vi "Mcp2210 Get Interrupt Count.vi"(8 "error in (no error)":errorcluster, 10 "Reset":bool, 11 "handle":i32) -> (0 "error out":errorcluster, 2 "pintCnt out":u32, 3 "handle out":i32)   [LabVIEW 2015, in "mcp2210.lvlib"]
doc: "Reads the event counter value. It may also reset the counter, depending on the reset\nparameter value. The function returns negative error code if something went wrong.\nNote: In order to have the MCP2210 record the number of external interrupt events,\nGP6 must be configured to have its dedicated function active.\nParameters:\nInputs:\n- void *handle - The pointer to the device handle. Cannot be NULL.\n- unsigned char reset - if set to 0, the counter is reset. Any other value has no effect.\nOutputs:\n- unsigned int *pintCnt - the value of the counter if the function returns E_SUCCESS.\nIn case of error *pintCnt is not modified.\nNote that the counter has 16bit resolution, so the maximum\nreturned value is 65535.\nCannot be NULL.\nReturns:\n- 0 for success: E_SUCCESS\n- negative error code: E_ERR_NULL, E_ERR_INVALID_HANDLE_VALUE\nE_ERR_UNKOWN_ERROR\nE_ERR_HID_TIMEOUT, E_ERR_HID_RW_FILEIO\nE_ERR_CMD_ECHO, E_ERR_CMD_FAILED\n\nMCP2210_DLL_UM_API int __stdcall Mcp2210_GetInterruptCount(void *handle, unsigned int *pintCnt, unsigned char reset);"
uses:
  <userlib>/mcp2210/mcp2210.lvlib
  <userlib>/mcp2210/mcp2210_dll_um_x86.dll
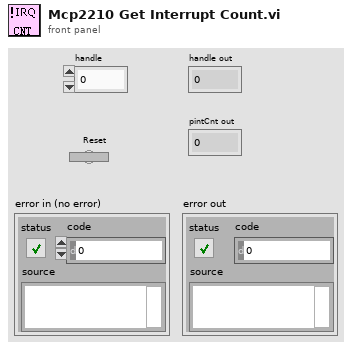
[diagram p1: front panel]
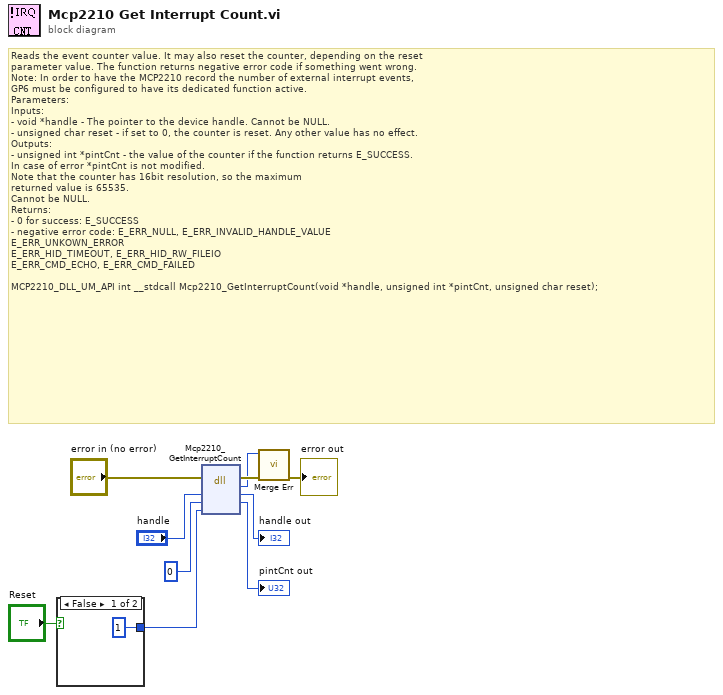
[diagram p0: block diagram]
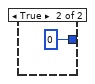
[diagram p2: hidden frame]
diagram:
  # "Reads the event counter value. It may also reset the counter, depending on the reset\nparameter value. The function returns negative error code if something went wrong.\nNote: In order to have the MCP2210 record the number of external interrupt events,\nGP6 must be configured to have its dedicated function active.\nParameters:\nInputs:\n- void *handle - The pointer to the device handle. Cannot be NULL.\n- unsigned char reset - if set to 0, the counter is reset. Any other value has no effect.\nOutputs:\n- unsigned int *pintCnt - the value of the counter if the function returns E_SUCCESS.\nIn case of error *pintCnt is not modified.\nNote that the counter has 16bit resolution, so the maximum\nreturned value is 65535.\nCannot be NULL.\nReturns:\n- 0 for success: E_SUCCESS\n- negative error code: E_ERR_NULL, E_ERR_INVALID_HANDLE_VALUE\nE_ERR_UNKOWN_ERROR\nE_ERR_HID_TIMEOUT, E_ERR_HID_RW_FILEIO\nE_ERR_CMD_ECHO, E_ERR_CMD_FAILED\n\nMCP2210_DLL_UM_API int __stdcall Mcp2210_GetInterruptCount(void *handle, unsigned int *pintCnt, unsigned char reset);"
  n1 = case shown="False" "Reset" {
    tunnel: [u8 1 ("reset") u8 0 ("reset")] -> w6
    frame False {
    }
    frame True {
    }
  }
  n2 = dll-call lib="D:/LabVIEW 2015/user.lib/mcp2210/mcp2210_dll_um_x86.*" fn="Mcp2210_GetInterruptCount"(error in="error in (no error)", "handle"="handle", "pintCnt"=u32 0, "reset"=w6) -> (error out=w5:errorcluster, "return type"=w4:i32, "handle"=→"handle out":i32, "pintCnt"=→"pintCnt out":u32)  [unwired: 3 in, 1 out]
  n3 = call <userlib>:"Merge Err.vi"("error in (no error)"=w5, "return type"=w4) -> ("error out"=→"error out":errorcluster)  [unwired: 9 in]
